vi "UI_test.vi"() -> ()   [LabVIEW 2017]
panel:
  out "output array":dbl[][](array[numeric])
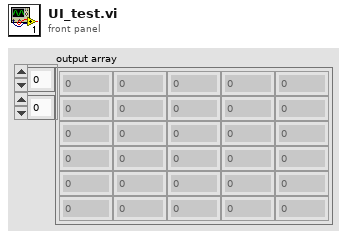
[diagram p1: front panel]
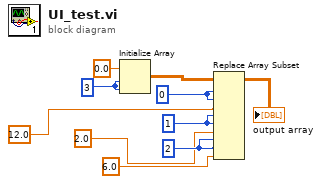
[diagram p0: block diagram]
diagram:
  w5 = 3 ("dimension size")
  w9 = 2 ("disabled index (row)")
  w10 = 1 ("disabled index (row)")
  w8 = 0 ("disabled index (row)")
  n1 = Initialize Array(0.0 ("element"), w5, w5) -> (w7:dbl[][])
  n2 = Replace Array Subset(array=w7, new element #1=12.0 ("new element/subarray"), index (row) #1=w8, index (col) #1=w8, new element #2=2.0 ("new element/subarray"), index (row) #2=w10, index (col) #2=w10, new element #3=6.0 ("new element/subarray"), index (row) #3=w9, index (col) #3=w9) -> (→"output array":dbl[][])
